vi "Example Program.vi"() -> ()   [LabVIEW 2012]
uses:
  <vilib>/DAQmx/write.llb/DAQmx Write.vi
  <vilib>/DAQmx/write.llb/DAQmx Write (Digital 1D Bool NChan 1Samp 1Line).vi
  <vilib>/DAQmx/configure/task.llb/DAQmx Clear Task.vi
  <vilib>/DAQmx/create/task.llb/DAQmx Create Task.vi
  <vilib>/DAQmx/configure/task.llb/DAQmx Start Task.vi
  <vilib>/DAQmx/create/channels.llb/DAQmx Create Virtual Channel.vi
  <vilib>/DAQmx/create/channels.llb/DAQmx Create Channel (DO-Digital Output).vi
  <vilib>/DAQmx/miscellaneous.llb/DAQmx Fill In Error Info.vi
panel:
  in  "Save Enable":bool
  in  "Save Interval":dbl=1.0 min=0.0 format="%<%H:%M:%S>t"
  out "Test Display":string="Mode: OFF  (Press Start to Begin)\r\r\r    "
  in  "STOP TEST":bool
  in  "START TEST":bool
  in  "File Name":string
  out "Graph Data":dbl[](array[numeric])
  out "Scaled Values":dbl[](array[numeric])
  in  "MAIN TAB":T1(tab)
  out "Graph":cluster{"t0":dbl, "dx":dbl, "Y Values":dbl[][]}(graph)
  out "9213 Error":errorcluster
  out "9205 Error":errorcluster
  out "9481 Error":errorcluster
  out "Scale Error":errorcluster
  out "Save Error":errorcluster
  in  "9213 Name":tag="9213"
  in  "9481 Name":tag="9481"
  in  "9205 Name":tag="9205"
  in  "9205 Config":T2={"Sample Rate [Hz]"=100.0, "Samples/Ch"=25, "Max Value [V]"=10.0, "Min Value [V]"=-10.0, "Rolling Average"=5, "HI/LO Trim [%]"=1.0, "Sample Timing Engine"=2} {"Sample Timing Engine" max=2; "Sample Rate [Hz]" min=0.0001 max=250000.0 format="%#_6p"; "Samples/Ch" min=1 step=1; "Max Value [V]" min=-10.0 max=10.0 format="%#_6p"; "Min Value [V]" min=-10.0 max=10.0 format="%#_6p"; "Rolling Average" min=1 step=1; "HI/LO Trim [%]" min=1.0 max=99.0}
  in  "9213 Config":T3={"Sample Rate [Hz]"=10.0, "Samples/Ch"=25, "Rolling Average"=5, "HI/LO Trim [%]"=1.0, "Sample Timing Engine"=2} {"Sample Timing Engine" max=2; "Sample Rate [Hz]" min=0.0001 max=75.0 format="%#_6p"; "Samples/Ch" min=1 step=1; "Rolling Average" min=1 step=1; "HI/LO Trim [%]" min=1.0 max=99.0}
  in  "Relay Control":bool[](array[boolean])=[FALSE, FALSE, FALSE, FALSE]
  out "Timer Elapsed":dbl[](array[numeric]) format="%<%H:%M:%S>t"
  in  "Timer Setpoints":dbl[](array[numeric])=[5.0, 0.0] format="%<%H:%M:%S>t"
  in  "Timer Enabled":bool[](array[boolean])=[TRUE, FALSE]
  out "MAIN Loop":i32
  out "EVENT Loop":i32
  in  "Save Folder Location":path
  out "File Path":path
  out "DAQ Loop":i32
  in  "Test Folder":path
  in  "Scale":T4={"Channel Select"=0, "Clear/Reset Scales"=FALSE, "Channel #"=["0", "1", "2"], "Scale Names"=["a", "b", "c"], "Set?"=[FALSE, FALSE, FALSE, FALSE, FALSE, FALSE], "HI/LO Setpoints"=[1.0, 0.0, 1.0, 0.0, 1.0, 0.0], "Units"=["vdc", "vdc", "vdc"], "HI/LO Signals"=[1.0, 0.0, 1.0, 0.0, 1.0, 0.0], "Slope/Intercept"=[1.0, 0.0, 1.0, 0.0, 1.0, 0.0], "IN/OUT Values"=[1.0, 1.0, 2.0, 2.0, 3.0, 3.0], "Sim Signals?"=FALSE, "Sim. Signal"=0.0} {"Sim. Signal" format="%#.3p"; "Channel Select" min=0 step=1; "Slope/Intercept" format="%#.3p"; "HI/LO Setpoints" format="%#.3p"; "IN/OUT Values" format="%#.3p"; "HI/LO Signals" format="%#.3p"}
  in  "Test Cluster":T5={"Load Test"=0, "New Test Name"="", "Test Description"="", "Step Select"=0, "Save Test"=FALSE, "Erase Test"=FALSE, "Max Steps"=15, "Loop Limit"=5, "Continue at Loop Limit?"=FALSE, "Step N"=2, "Test Array (Standard)"=[{"Step Number"=0, "Step Description"="Step Description", "Step Time Target"=10.0, "Step Time Unit"=0, "Step End Action"=0}], "Test Array (Custom)"=[{"Custom Actions"=0, "ch0"=FALSE, "ch1"=FALSE, "ch2"=FALSE, "ch3"=FALSE}]} {"Test Array (Custom)"."Custom Actions" items=["None", "Measure Signal", "Display Plot", "Save to File"]; "Test Array (Standard)"."Step End Action" items=["Go to Next Step", "Loop to Step 0", "Loop to Step N", "Stop Test Mode", "Stop Program"]; "Test Array (Standard)"."Step Time Unit" items=["sec", "min", "hr"]; "Test Array (Standard)"."Step Time Target" min=0.01 format="%#.2f"; "Test Array (Standard)"."Step Number" min=0 step=1; "Load Test" items=["Example1"]; "Step Select" step=1}
  in  "EXIT":bool
  in  "ECOLAB BUTTON":bool=TRUE
  # "Template LabVIEW Program"
  # "Created by Blake Otting  July 2013"
  # "Last Updated 8-5-13"
  # "9205 Configuration"
  # "9213 Configuration"
  # "Graph Update"
  # "HH:MM:SS"
  # "Not Used"
  # "HH:MM:SS"
  # "Ch.\n#"
  # "Scale\nName"
  # "Set\nValues?"
  # "Channel\nSelect"
  # "Scaled"
  # "Pre-Scaled"
  # "Scaling Result"
  # "Values"
  # "Units"
  # "Values"
  # "HI"
  # "Slope"
  # "IN"
  # "LO"
  # "Intercept"
  # "OUT"
  # "HI"
  # "Slope"
  # "IN"
  # "LO"
  # "Intercept"
  # "OUT"
  # "HI"
  # "Slope"
  # "IN"
  # "LO"
  # "Intercept"
  # "OUT"
  # "HI"
  # "Slope"
  # "IN"
  # "LO"
  # "Intercept"
  # "OUT"
  # "9481 Relay"
  # "Custom Action"
  # "Scroll"
  # "Step"
  # "Description"
  # "Time Target"
  # "End Action"
  # "0"
  # "1"
  # "2"
  # "3"
  # "Total #\nof Steps"
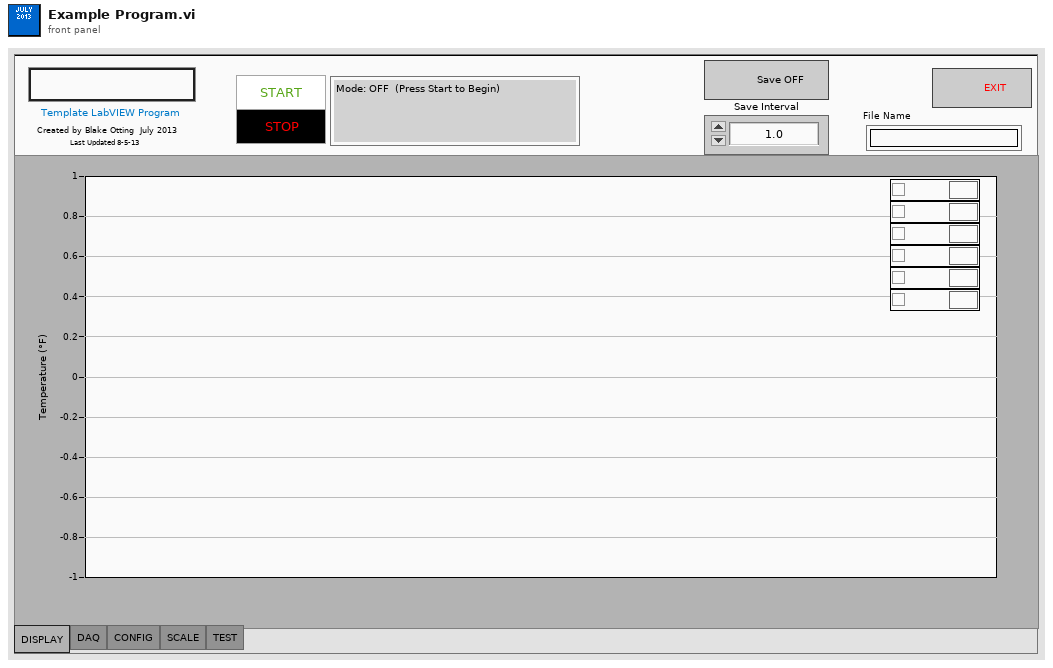
[diagram p1: front panel]
types:
  T1 = enum32{"DISPLAY", "DAQ", "CONFIG", "SCALE", "TEST"}
  T2 = cluster{"Sample Rate [Hz]":dbl, "Samples/Ch":i32, "Max Value [V]":dbl, "Min Value [V]":dbl, "Rolling Average":i32, "HI/LO Trim [%]":dbl, "Sample Timing Engine":u32}
  T3 = cluster{"Sample Rate [Hz]":dbl, "Samples/Ch":i32, "Rolling Average":i32, "HI/LO Trim [%]":dbl, "Sample Timing Engine":u32}
  T4 = cluster{"Channel Select":i32, "Clear/Reset Scales":bool, "Channel #":string[], "Scale Names":string[], "Set?":bool[], "HI/LO Setpoints":dbl[], "Units":string[], "HI/LO Signals":dbl[], "Slope/Intercept":dbl[], "IN/OUT Values":dbl[], "Sim Signals?":bool, "Sim. Signal":dbl}
  T5 = cluster{"Load Test":u16, "New Test Name":string, "Test Description":string, "Step Select":u16, "Save Test":bool, "Erase Test":bool, "Max Steps":u16, "Loop Limit":u16, "Continue at Loop Limit?":bool, "Step N":u16, "Test Array (Standard)":cluster{"Step Number":i32, "Step Description":string, "Step Time Target":dbl, "Step Time Unit":u16, "Step End Action":u16}[], "Test Array (Custom)":cluster{"Custom Actions":u16, "ch0":bool, "ch1":bool, "ch2":bool, "ch3":bool}[]}
  T6 = cluster{"Custom Actions":u16, "ch0":bool, "ch1":bool, "ch2":bool, "ch3":bool}
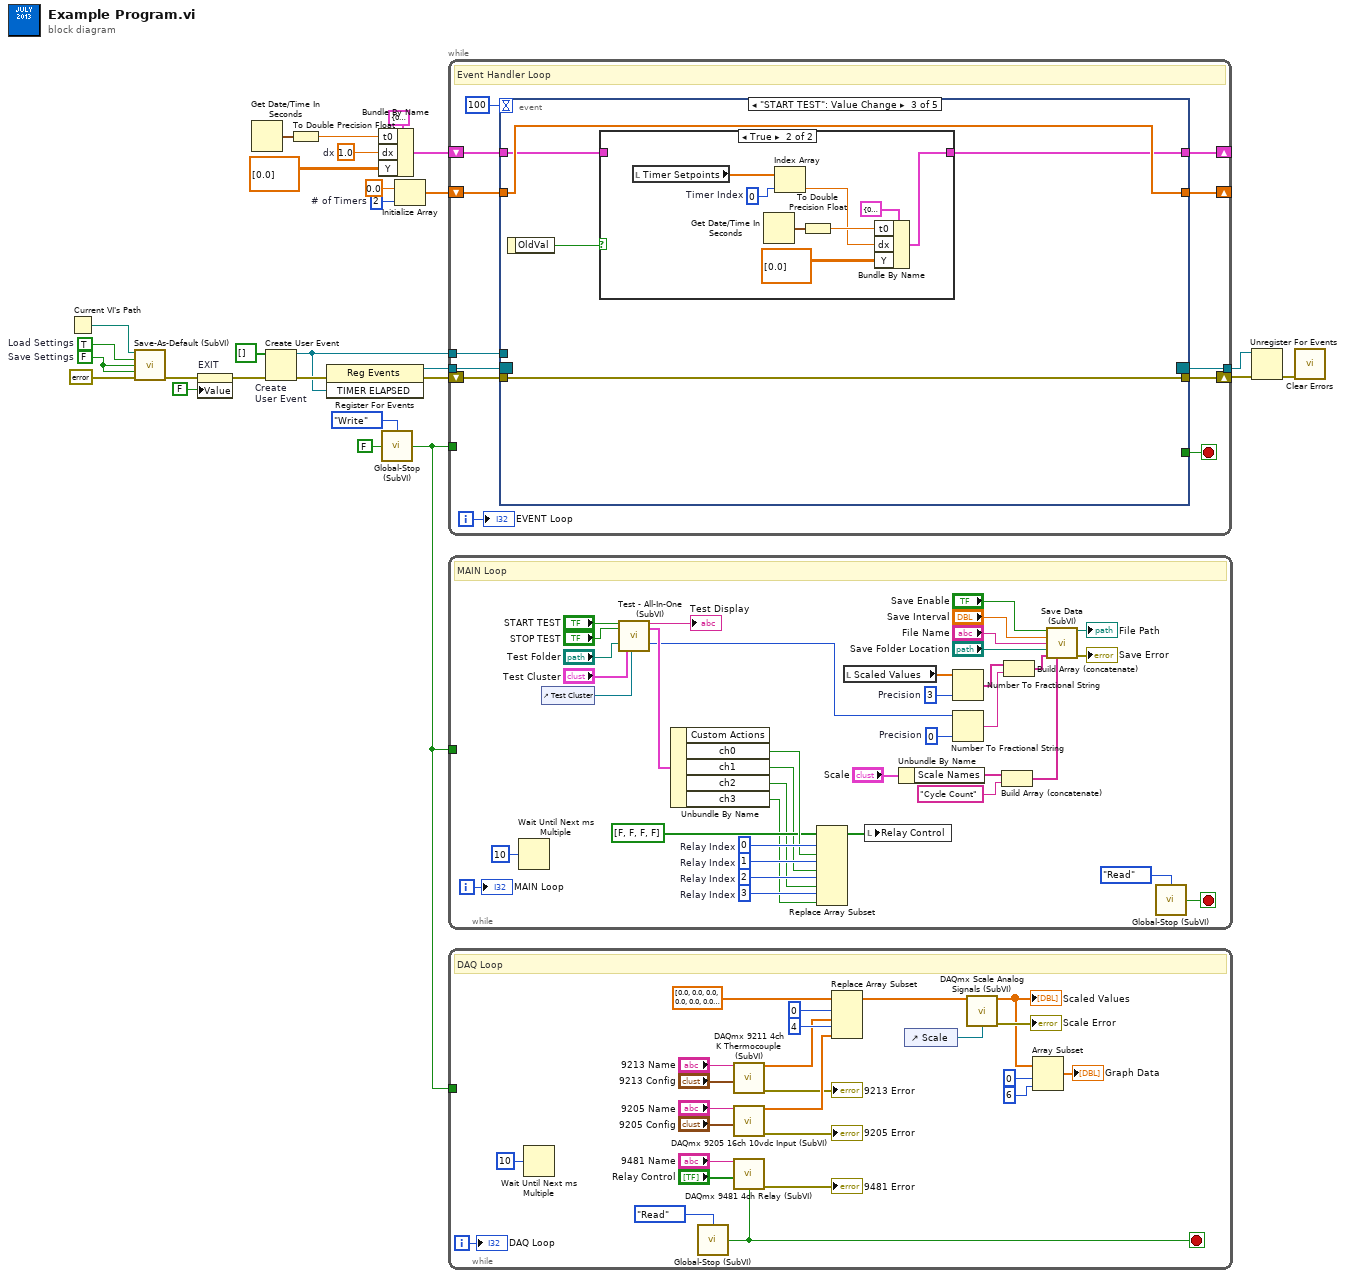
[diagram p0: block diagram]
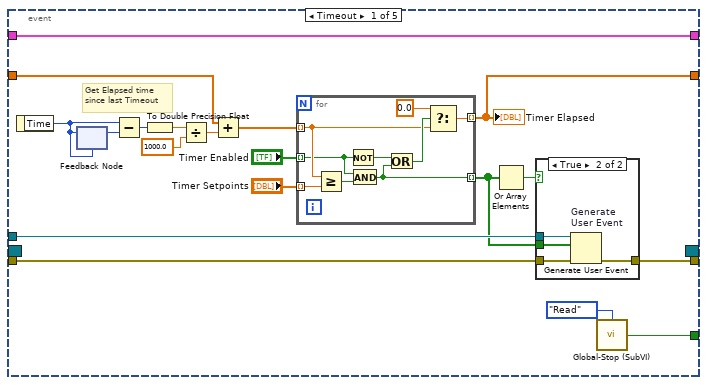
[diagram p2: hidden frame]
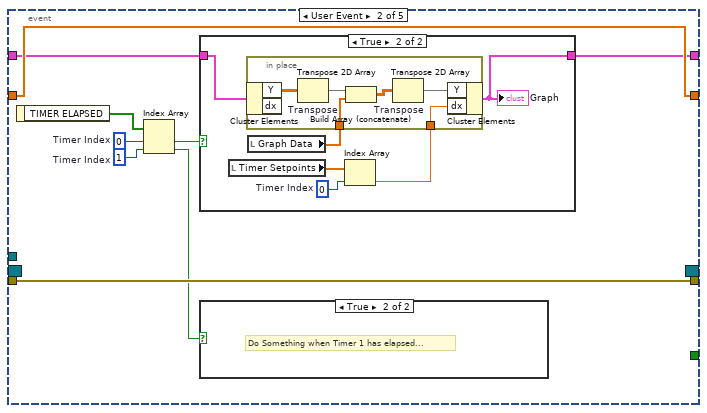
[diagram p4: hidden frame]
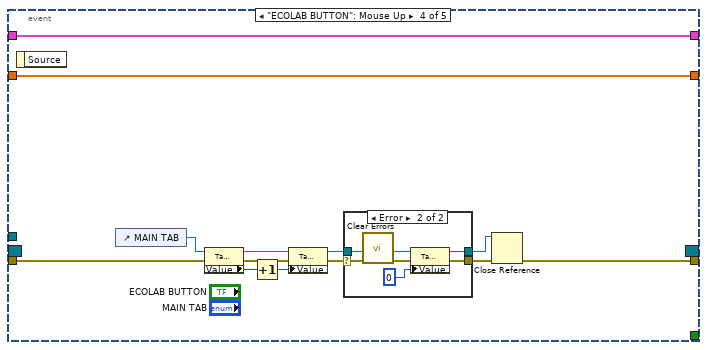
[diagram p8: hidden frame]
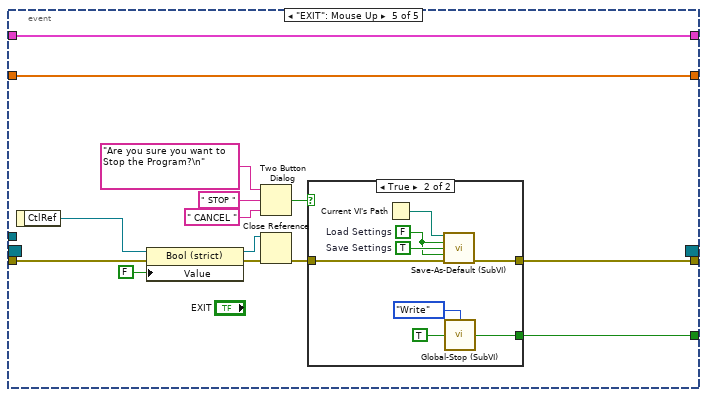
[diagram p10: hidden frame]
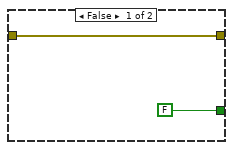
[diagram p11: hidden frame]
diagram:
  w3 = 1.0  # dx
  w12 = 2  # # of Timers
  w25 = FALSE  # Save Settings
  w24 = TRUE  # Load Settings
  n1 = Current VI's Path() -> (path=w7:path)
  n2 = call "Save-As-Default (SubVI).vi"("Current VI's Path"=w7, "Load Settings"=w24, "Save Settings"=w25, "Save and Exit"=w25, "Error IN"=errorcluster {"status"=FALSE, "code"=0, "source"=""}) -> ("Save as Default Error"=w22:errorcluster)  [unwired: 10 in]
  n3 = property on="EXIT" class="Bool (strict)"(error in=w22, "Value"=FALSE) -> (error out=w17:errorcluster)  [unwired: 1 in, 1 out]
  n4 = Get Date/Time In Seconds() -> (seconds since 1Jan1904=w6:timestamp)
  n5 = Create User Event "Create\nUser Event"(user event datatype=bool[] [] ("TIMER ELAPSED"), error in=w17) -> (user event=w14:refnum<user-event>, error out=w16:errorcluster)
  n6 = To Double Precision Float(number=w6) -> (double precision float=w4:dbl)
  n7 = register-events(error in=w16, w14) -> (reference out=w19:refnum<event-registration>, error out=w15:errorcluster)  [unwired: 1 in]
  n8 = Bundle By Name(cluster=cluster{"t0":dbl, "dx":dbl, "Y":dbl[][]} {"t0"=0.0, "dx"=0.0, "Y"=[]} ("Graph"), "t0"=w4, "dx"=w3, "Y"=dbl[][] [[0.0]] ("Y Values")) -> (w1:cluster{"t0":dbl, "dx":dbl, "Y":dbl[][]})
  n9 = call "Global-Stop (SubVI).vi"("Mode (Read)"=enum16{"Read", "Write"}."Write", "IN"=FALSE) -> ("OUT"=w23:bool)  [unwired: 2 in]
  n10 = Initialize Array(0.0, w12) -> (w11:dbl[])
  n11 = while {
    shift-right: [w33] -> _
    shift-left: w11 -> [w38]
    shift-right: [w37] -> w9
    shift-left: w15 -> [w35]
    tunnel: w23 -> [_]
    tunnel: w19 -> [w32]
    tunnel: w14 -> [w31]
    tunnel: [w30] -> w10
    shift-right: [w28] -> _
    shift-left: w1 -> [w29]
    i -> [w34]
    stop <- w36 stop-if-true
    # "Event Handler Loop"
    n12 = event shown="[2] \"START TEST\": Value Change" {
      selector: w32 -> [_ _ _ _ _]
      dyn-events: [_ _ _ _ _] -> w30
      timeout: 100 -> [_ _ _ _ _]
      tunnel: w38 -> [w52 w77 w99 w110 w137]
      tunnel: [w47 w81 w98 w111 w139] -> w37
      tunnel: [w50 _ _ _ w138] -> w36
      tunnel: w35 -> [w48 w81 w98 w112 w134]
      tunnel: [w41 w77 w99 w110 w137] -> w33
      tunnel: w31 -> [w49 _ _ _ _]
      tunnel: w29 -> [w40 w74 w96 w109 w130]
      tunnel: [w40 w73 w97 w109 w130] -> w28
      event Timeout {
        # "Get Elapsed time\nsince last Timeout"
        n13 = event-data() -> ("Time"=w53:u32)  [unwired: 1 in]
        n14 = feedback #1(w53) -> (w56:u32)
        n15 = feedback-in #1(w53) -> ()
        n16 = Subtract(x=w53, y=w56) -> (x-y=w55:u32)
        n17 = To Double Precision Float(number=w55) -> (double precision float=w57:dbl)
        n18 = Divide(x=w57, y=1000.0) -> (x/y=w54:dbl)
        n19 = Add(x=w52, y=w54) -> (x+y=w42:dbl[])
        n20 = for {
          tunnel: w42 -> [w68] mode=indexing
          tunnel: "Timer Enabled" -> [w65] mode=indexing
          tunnel: "Timer Setpoints" -> [w72] mode=indexing
          tunnel: [w71] -> w41 mode=indexing
          tunnel: [w66] -> w43 mode=indexing
          n21 = Greater Or Equal?(x=w68, y=w72) -> (x >= y?=w64:bool)
          n22 = Not(x=w65) -> (.not. x?=w67:bool)
          n23 = And(x=w65, y=w64) -> (x .and. y?=w66:bool)
          n24 = Or(x=w67, y=w66) -> (x .or. y?=w70:bool)
          n25 = Select(t=0.0, s=w70, f=w68) -> (s? t:f=w71:dbl)
        }
        "Timer Elapsed" <- w41
        n26 = Or Array Elements(Boolean array=w43) -> (logical OR=w44:bool)
        n27 = case shown="True" w44 {
          tunnel: w49 -> [_ w63]
          tunnel: w48 -> [w59 w62]
          tunnel: [w59 w61] -> w47
          tunnel: w43 -> [_ w60]
          frame False {
          }
          frame True {
            n28 = Generate User Event "Generate\nUser Event"(user event=w63, event data cluster=w60, error in=w62) -> (error out=w61:errorcluster)  [unwired: 1 out]
          }
        }
        n29 = call "Global-Stop (SubVI).vi"("Mode (Read)"=enum16{"Read", "Write"}."Read") -> ("OUT"=w50:bool)  [unwired: 3 in]
      }
      event User Event {
        w76 = 1  # Timer Index
        w78 = 0  # Timer Index
        n30 = event-data() -> ("TIMER ELAPSED"=w80:bool[])  [unwired: 1 in]
        n31 = Index Array(array=w80, index #1=w78, index #2=w76) -> (element #1=w79:bool, element #2=w75:bool)
        n32 = case shown="True" w79 {
          tunnel: w74 -> [w82 w88]
          tunnel: [w82 w87] -> w73
          frame False {
          }
          frame True {
            w86 = 0  # Timer Index
            n33 = local read "Timer Setpoints"() -> (w85:dbl[])
            n34 = local read "Graph Data"() -> (w83:dbl[])
            n35 = Index Array(array=w85, index=w86) -> (element=w84:dbl)
            n36 = in-place {
              in-place-border: w83 -> [w90]
              in-place-border: w84 -> [w89]
              n37 = in-place-cluster #2(w88) -> ("Y"=w92:dbl[][])  [unwired: 1 out]
              n38 = Transpose 2D Array "Transpose"(2D array=w92) -> (transposed array=w94:dbl[][])
              n39 = Build Array (concatenate)(w94, w90) -> (w93:dbl[][])
              n40 = Transpose 2D Array "Transpose"(2D array=w93) -> (transposed array=w91:dbl[][])
              n41 = in-place-cluster #2("Y"=w91, "dx"=w89) -> (w87:cluster{"t0":dbl, "dx":dbl, "Y":dbl[][]})
            }
            "Graph" <- w87
          }
        }
        n42 = case shown="True" w75 {
          frame False {
          }
          frame True {
            # "Do Something when Timer 1 has elapsed..."
          }
        }
      }
      event "START TEST": Value Change {
        n43 = event-data() -> ("OldVal"=w95:bool)  [unwired: 1 in]
        n44 = case shown="True" w95 {
          tunnel: [w100 w104] -> w97
          tunnel: w96 -> [w100 _]
          frame False {
          }
          frame True {
            w103 = 0  # Timer Index
            n45 = local read "Timer Setpoints"() -> (w102:dbl[])
            n46 = Get Date/Time In Seconds() -> (seconds since 1Jan1904=w108:timestamp)
            n47 = Index Array(array=w102, index=w103) -> (element=w101:dbl)
            n48 = To Double Precision Float(number=w108) -> (double precision float=w106:dbl)
            n49 = Bundle By Name(cluster=cluster{"t0":dbl, "dx":dbl, "Y":dbl[][]} {"t0"=0.0, "dx"=0.0, "Y"=[]} ("Graph"), "t0"=w106, "dx"=w101, "Y"=dbl[][] [[0.0]] ("Y Values")) -> (w104:cluster{"t0":dbl, "dx":dbl, "Y":dbl[][]})
          }
        }
      }
      event "ECOLAB BUTTON": Mouse Up {
        n50 = event-data() -> ()  [unwired: 1 in, 1 out]
        n51 = control-ref of="MAIN TAB"() -> (w121:refnum<vi>)
        n52 = property class="TabCtl (strict)"(reference=w121, error in=w112) -> (reference out=w119:refnum<vi>, error out=w117:errorcluster, "Value"=w120:T1)
        n53 = Increment(x=w120) -> (x+1=w118:T1)
        n54 = property class="TabCtl (strict)"(reference=w119, error in=w117, "Value"=w118) -> (reference out=w115:refnum<vi>, error out=w116:errorcluster)
        n55 = case shown="Error" w116 {
          selector: w116 -> [w122 w127]
          tunnel: w115 -> [w123 w129]
          tunnel: [w122 w126] -> w114
          tunnel: [w123 w125] -> w113
          frame No Error {
          }
          frame Error {
            n56 = call <vilib>:"Clear Errors.vi"("error in (no error)"=w127) -> ("error out"=w124:errorcluster)  [unwired: 6 in]
            n57 = property class="TabCtl (strict)"(reference=w129, error in=w124, "Value"=0) -> (reference out=w125:refnum<vi>, error out=w126:errorcluster)
          }
        }
        n58 = Close Reference(reference=w113, error in (no error)=w114) -> (error out=w111:errorcluster)
      }
      event "EXIT": Mouse Up {
        n59 = event-data() -> ("CtlRef"=w136:refnum<vi>)  [unwired: 1 in]
        n60 = property class="Bool (strict)"(reference=w136, error in=w134, "Value"=FALSE) -> (reference out=w133:refnum<vi>, error out=w132:errorcluster)
        n61 = Two Button Dialog(message="Are you sure you want to Stop the Program?\n", 1:" CANCEL " ("F button name (\"Cancel\")"), 2:" STOP ") -> (T button?=w140:bool)
        n62 = Close Reference(reference=w133, error in (no error)=w132) -> (error out=w131:errorcluster)
        n63 = case shown="True" w140 {
          tunnel: [w144 w153] -> w139
          tunnel: [FALSE w150] -> w138
          tunnel: w131 -> [w144 w148]
          frame False {
          }
          frame True {
            w147 = TRUE  # Save Settings
            w146 = FALSE  # Load Settings
            n64 = Current VI's Path() -> (path=w149:path)
            n65 = call "Save-As-Default (SubVI).vi"("Current VI's Path"=w149, "Load Settings"=w146, "Save Settings"=w147, "Save and Exit"=w146, "Error IN"=w148) -> ("Save as Default Error"=w153:errorcluster)  [unwired: 10 in]
            n66 = call "Global-Stop (SubVI).vi"("Mode (Read)"=enum16{"Read", "Write"}."Write", "IN"=TRUE) -> ("OUT"=w150:bool)  [unwired: 2 in]
          }
        }
      }
    }
    "EVENT Loop" <- w34
  }
  n67 = while {
    tunnel: w23 -> [_]
    i -> [w191]
    stop <- w190 stop-if-true
    w173 = i16 0  # Precision
    w176 = 3  # Relay Index
    w177 = 2  # Relay Index
    w178 = 1  # Relay Index
    w179 = 0  # Relay Index
    w187 = i16 3  # Precision
    # "MAIN Loop"
    n68 = Wait Until Next ms Multiple(millisecond multiple=u32 10) -> ()  [unwired: 1 out]
    n69 = control-ref of="Test Cluster"() -> (w160:refnum<vi>)
    n70 = call "Test - All-In-One (SubVI).vi"("START TEST"="START TEST", "STOP TEST"="STOP TEST", "Test Folder"="Test Folder", "Test Cluster"="Test Cluster", "Test Cluster Ref"=w160) -> ("Test Display"=→"Test Display":string, "Test Output"=w162:T6, "Loop Number"=w159:u16)  [unwired: 7 in, 5 out]
    n71 = Unbundle By Name(w162) -> ("ch0"=w158:bool, "ch1"=w156:bool, "ch2"=w155:bool, "ch3"=w154:bool)  [unwired: 1 out]
    n72 = Replace Array Subset(array=bool[] [FALSE, FALSE, FALSE, FALSE] ("Relay Control"), new element #1=w158, index #1=w179, new element #2=w156, index #2=w178, new element #3=w155, index #3=w177, new element #4=w154, index #4=w176) -> (w175:bool[])
    n73 = local read "Scaled Values"() -> (w188:dbl[])
    n74 = local write "Relay Control"(w175) -> ()
    n75 = Unbundle By Name("Scale") -> ("Scale Names"=w169:string[])
    n76 = Number To Fractional String(number=w188, precision (6)=w187) -> (F-format string=w172:string[])  [unwired: 2 in]
    n77 = Number To Fractional String(number=w159, precision (6)=w173) -> (F-format string=w171:string)  [unwired: 2 in]
    n78 = Build Array (concatenate)(w169, "Cycle Count") -> (w167:string[])
    n79 = Build Array (concatenate)(w172, w171) -> (w170:string[])
    n80 = call "Save Data (SubVI).vi"("Save Enable"="Save Enable", "Save Interval [sec]"="Save Interval", "File Name"="File Name", "Folder Location"="Save Folder Location", "Data Array (Row)"=w170, "Column Header Array"=w167) -> ("File Path"=→"File Path":path, "Save Error"=→"Save Error":errorcluster)  [unwired: 7 in, 1 out]
    n81 = call "Global-Stop (SubVI).vi"("Mode (Read)"=enum16{"Read", "Write"}."Read") -> ("OUT"=w190:bool)  [unwired: 3 in]
    "MAIN Loop" <- w191
  }
  n82 = while {
    tunnel: w23 -> [_]
    i -> [w216]
    stop <- w199 stop-if-true
    # "DAQ Loop"
    n83 = Wait Until Next ms Multiple(millisecond multiple=u32 10) -> ()  [unwired: 1 out]
    n84 = call "Global-Stop (SubVI).vi"("Mode (Read)"=enum16{"Read", "Write"}."Read") -> ("OUT"=w199:bool)  [unwired: 3 in]
    n85 = call "DAQmx 9211 4ch K Thermocouple (SubVI).vi"("9211 Name"="9213 Name", "9211 Config"="9213 Config") -> ("Measurements"=w196:dbl[], "9211 Error"=→"9213 Error":errorcluster)  [unwired: 12 in]
    n86 = call "DAQmx 9205 16ch 10vdc Input (SubVI).vi"("9205 Name"="9205 Name", "9205 Config"="9205 Config") -> ("Measurements"=w205:dbl[], "9205 Error"=→"9205 Error":errorcluster)  [unwired: 12 in]
    n87 = call "DAQmx 9481 4ch Relay (SubVI).vi"("9481 Name"="9481 Name", "Relay Control"="Relay Control", "Stop Program"=w199) -> ("9481 Error"=→"9481 Error":errorcluster)  [unwired: 12 in]
    n88 = Replace Array Subset(array=dbl[] [0.0, 0.0, 0.0, 0.0, 0.0, 0.0, 0.0, 0.0, 0.0, 0.0, 0.0, 0.0, 0.0, 0.0, 0.0, 0.0, 0.0, 0.0, 0.0, 0.0], new element #1=w196, index #1=0, new element #2=w205, index #2=4) -> (w203:dbl[])
    n89 = control-ref of="Scale"() -> (w214:refnum<vi>)
    n90 = call "DAQmx Scale Analog Signals (SubVI).vi"("Measured Signals"=w203, "Scale Reference"=w214) -> ("Scaled Values"=w195:dbl[], "Scale Error"=→"Scale Error":errorcluster)  [unwired: 12 in]
    "Scaled Values" <- w195
    n91 = Array Subset(array=w195, index=0, length=6) -> (→"Graph Data":dbl[])
    "DAQ Loop" <- w216
  }
  n92 = Unregister For Events(event registration refnum=w10, error in=w9) -> (error out=w8:errorcluster)
  n93 = call <vilib>:"Clear Errors.vi"("error in (no error)"=w8) -> ()  [unwired: 6 in, 1 out]
